vi "WriteDarkColor.vi"(4 "error in (no error)":errorcluster, 5 "Value":u32(colorbox), 6 "Container State":T3, 7 "Display State In":T1) -> (0 "error out":errorcluster, 3 "Display State Out":T1)   [LabVIEW 2013, in "BarCodes.lvlib" / "Barcode.xctl"]
uses:
  Barcode.xctl
  <vilib>/_xctls/Container State.ctl
  State.ctl
  BarcodeType.ctl
  <vilib>/_xctls/XControlSupport.lvlib
  BarCodes.lvlib
panel:
  # "Replace the Value Control below with a Control of desired type.\nDo not remove this Control or the others from the connector pane.\nDo not change the connector pane pattern.\nThe Value control should always be the third terminal from top on the input side in the connector pane."
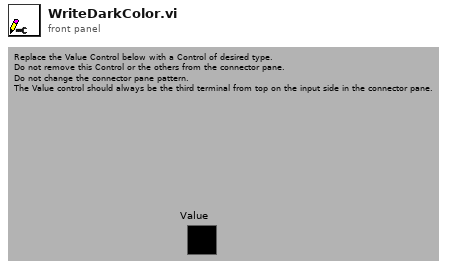
[diagram p1: front panel]
types:
  T1 = typedef "BarCodes.lvlib/Barcode.xctl/State.ctl" = cluster{"BarcodeType":T2, "Scale":u8, "Dark Color":u32, "Light Color":u32}
  T2 = typedef "BarCodes.lvlib/BarcodeType.ctl" = enum16{"EAN-13", "UPC", "Code 39 (3 of 9)", "Code 128"}
  T3 = typedef "XControlSupport.lvlib/Container State.ctl" = cluster{"Indicator?":bool, "Run Mode?":bool, " Refnum":refnum<vi>}
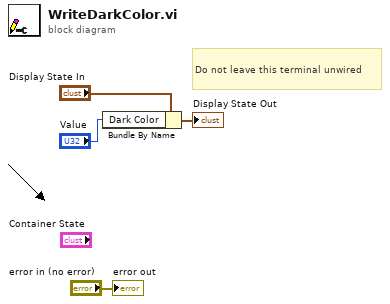
[diagram p0: block diagram]
diagram:
  # "Do not leave this terminal unwired"
  n1 = Bundle By Name(cluster="Display State In", "Dark Color"="Value") -> (→"Display State Out":T1)
  "error out" <- "error in (no error)"
